vi "Get unitary matrix.vi"(8 "error in (no error)":errorcluster, 11 "G-UE in":refnum<class "G-UE.lvclass">) -> (0 "error out":errorcluster, 2 "Unitary matrix":T1, 3 "G-UE out":refnum<class "G-UE.lvclass">)   [LabVIEW 2016, in "G-UE.lvclass"]
uses:
  G-UE.lvclass
  <vilib>/Analysis/Matrix/Datatypes/ComplexMatrix.ctl
  G-UE.lvclass/G-UE.ctl
  <vilib>/Analysis/Matrix/NI_Matrix.lvlib
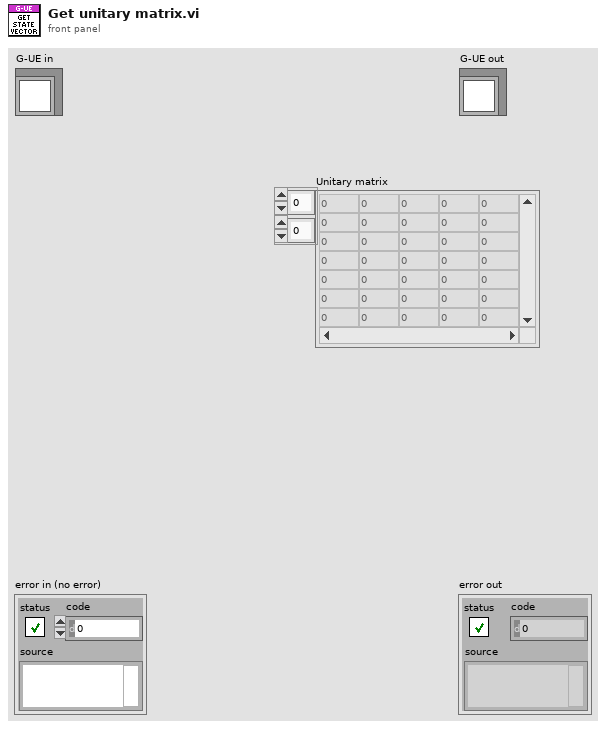
[diagram p1: front panel]
types:
  T1 = typedef "NI_Matrix.lvlib/ComplexMatrix.ctl" = cdb[][]
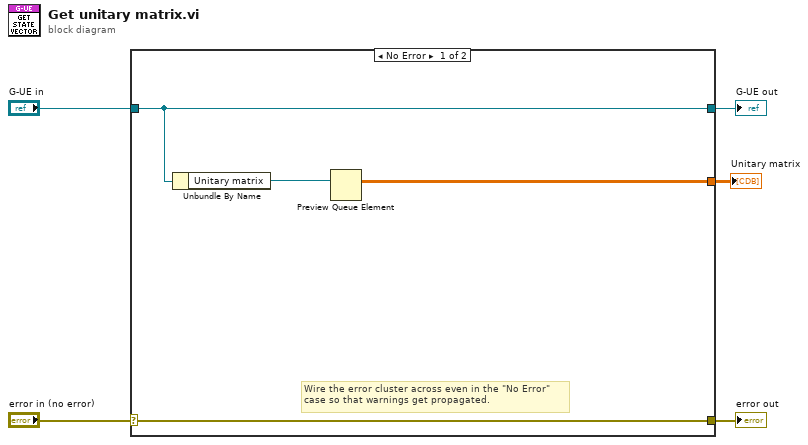
[diagram p0: block diagram]
diagram:
  n1 = case shown="No Error" "error in (no error)" {
    selector: "error in (no error)" -> [w9 w11]
    tunnel: [w9 w11] -> w4
    tunnel: [w8 w10] -> w2
    tunnel: "G-UE in" -> [w8 w10]
    tunnel: [w6 _] -> w1
    frame No Error {
      # "Wire the error cluster across even in the \"No Error\"\ncase so that warnings get propagated."
      n2 = Unbundle By Name(w8) -> ("Unitary matrix"=w7:refnum<queue>)
      n3 = Preview Queue Element(queue=w7) -> (element=w6:T1)  [unwired: 2 in, 3 out]
    }
    frame Error {
    }
  }
  "error out" <- w4
  "G-UE out" <- w2
  "Unitary matrix" <- w1
